vi "Driving with the Limelight.vi"() -> (0 "TurnCommand":dbl(knob)=nan scale=-1.0..1.0, 1 "SpeedCommand":dbl(knob)=-0.0 scale=0.0..1.0, 3 "TargetValid":bool)   [LabVIEW 2019]
uses:
  Framework/Robot Global Data.vi
panel:
  in  "SteeringK":dbl(slide)=0.025362318840579712 min=0.0 max=0.25 step=0.01 scale=0.0..0.25
  in  "MinSteerCommand":dbl(slide)=0.2717391304347826 min=0.0 max=0.5 step=0.05 scale=0.0..0.5
  in  "AimDeadband":dbl min=0.0 max=10.0 step=0.25
  in  "Limelight Goal Area":dbl(slide)=14.872262773722628 min=0.1 max=25.0 step=0.25 scale=0.0..25.0
  in  "DriveK":dbl(slide)=0.26277372262773724 min=0.0 max=1.0 step=0.05 scale=0.0..1.0
  in  "MaxDrive":dbl(slide)=0.6824817518248175 min=0.0 max=1.0 step=0.01 scale=0.0..1.0
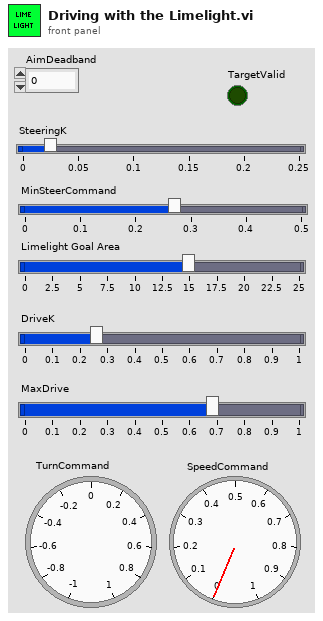
[diagram p1: front panel]
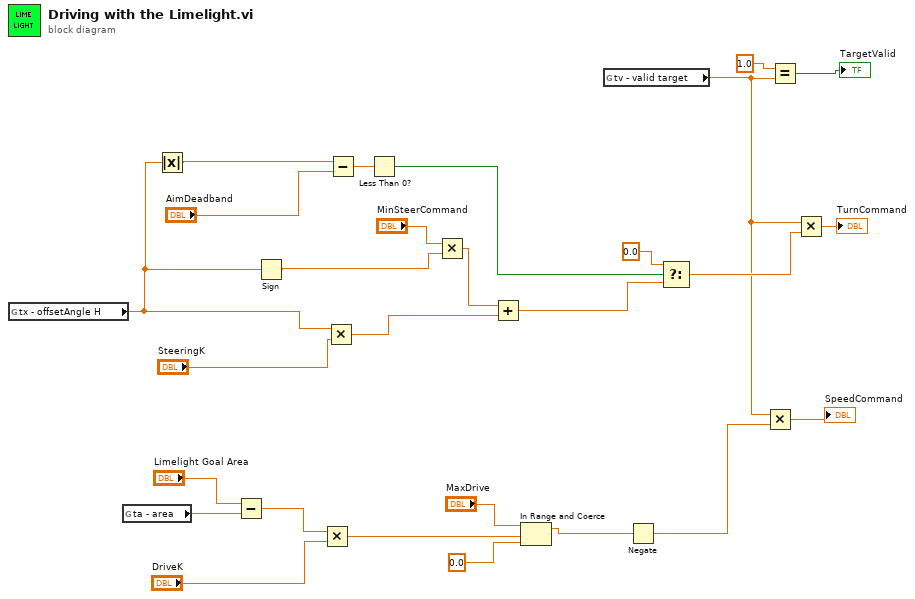
[diagram p0: block diagram]
diagram:
  n1 = global read "Robot Global Data.vi" "tx - offsetAngle H"() -> (w3:dbl)
  n2 = global read "Robot Global Data.vi" "ta - area"() -> (w2:dbl)
  n3 = Absolute Value(x=w3) -> (abs(x)=w23:dbl)
  n4 = Subtract(x="Limelight Goal Area", y=w2) -> (x-y=w13:dbl)
  n5 = Sign(1:w3) -> (0:w16:dbl)
  n6 = Multiply(x=w13, y="DriveK") -> (x*y=w12:dbl)
  n7 = Multiply(x=w3, y="SteeringK") -> (x*y=w20:dbl)
  n8 = Subtract(x=w23, y="AimDeadband") -> (x-y=w25:dbl)
  n9 = Less Than 0?(x=w25) -> (x < 0?=w26:bool)
  n10 = Multiply(x="MinSteerCommand", y=w16) -> (x*y=w22:dbl)
  n11 = Add(x=w22, y=w20) -> (x+y=w6:dbl)
  n12 = In Range and Coerce(upper limit="MaxDrive", x=w12, lower limit=0.0) -> (coerced(x)=w8:dbl)  [unwired: 1 out]
  n13 = global read "Robot Global Data.vi" "tv - valid target"() -> (w1:dbl)
  n14 = Negate(x=w8) -> (-x=w7:dbl)
  n15 = Select(t=0.0, s=w26, f=w6) -> (s? t:f=w19:dbl)
  n16 = Multiply(x=w1, y=w7) -> (x*y=→"SpeedCommand":dbl)
  n17 = Equal?(x=1.0, y=w1) -> (x = y?=→"TargetValid":bool)
  n18 = Multiply(x=w1, y=w19) -> (x*y=→"TurnCommand":dbl)
